vi "4Pi 4Pi Modes Control.vi"(7 "Calling VI Ref":refnum<vi>) -> ()   [LabVIEW 2016]
uses:
  <vilib>/Analysis/NI_AALBase.lvlib
  <vilib>/Utility/file.llb/Read Delimited Spreadsheet (DBL).vi
  <vilib>/Utility/miscctls.llb/LVPointTypeDef.ctl
  <vilib>/Analysis/baseanly.llb/Mean (DBL).vi
  4Pi 4Pi Modes - Controls/4Pi 4Pi Modes - Standard Action.ctl
  <vilib>/Utility/file.llb/Write Delimited Spreadsheet (DBL).vi
  4Pi 4Pi Modes - Controls/4Pi 4Pi Modes - Mirror Modes.ctl
panel:
  out "Pixel Map (-1 to 1) 2":dbl[][](graph)
  in  "Scan Modes":bool
  in  "Astig On/Off":bool
  in  "Load Astig":bool
  in  "Active Mirror":enum32{"Mirror 1", "Mirror 2"}(radio)
  in  "Clear Modes":bool
  in  "Mirror Modes":T1
  in  "Load Modes":bool
  in  "Save Modes":bool
  in  "Load Flat":bool
  in  "Apply Zero":bool
  in  "Load V Map":bool
  in  "Save V Map":bool
  in  "Apply Flat":bool
  in  "Center Bias":bool
  in  "Quit":bool
  out "Pixel Map (-1 to 1)":dbl[][](graph)
  # "Mode"
  # "Amount (nm)"
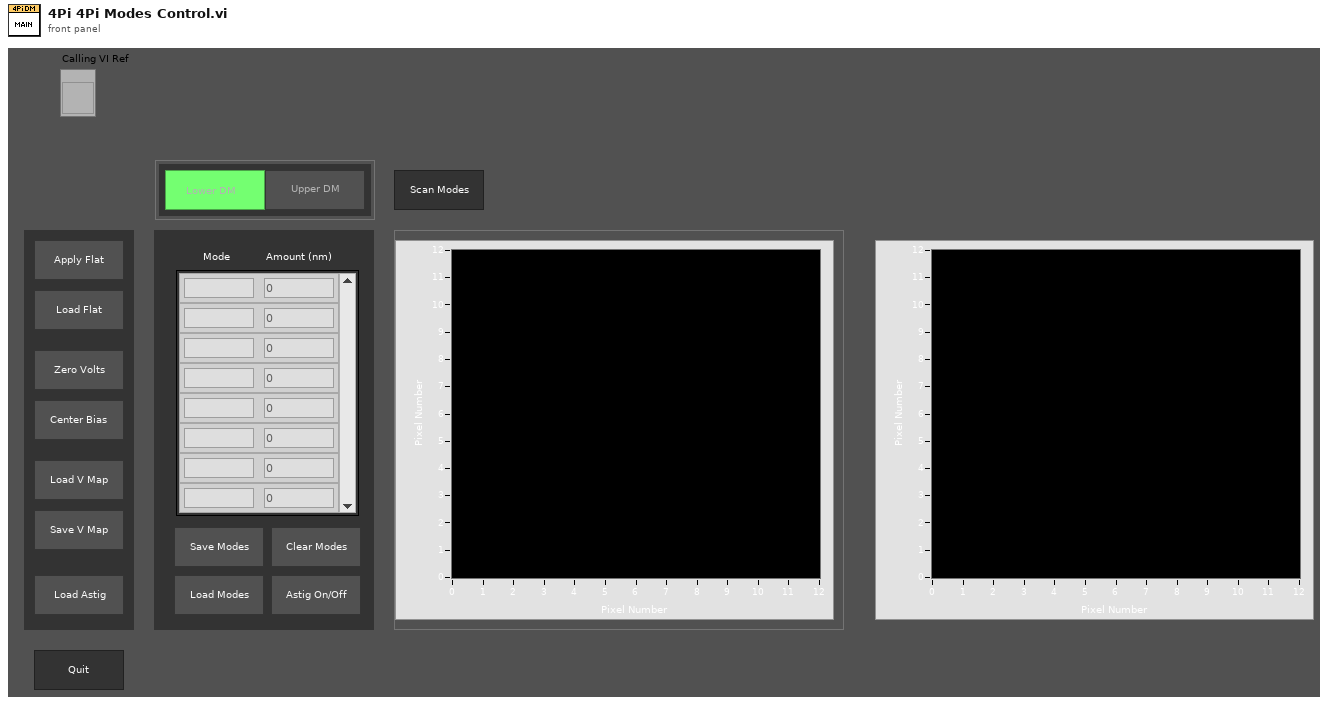
[diagram p1: front panel]
types:
  T1 = typedef "4Pi 4Pi Modes - Mirror Modes.ctl" = cluster{"Mode":string, "Amplitude":dbl}[]
  T2 = enum16{"Always On", "Always Off", "Off While Running"}
  T3 = typedef "LVPointTypeDef.ctl" = cluster{"Horizontal":i16, "Vertical":i16}
  T4 = typedef "4Pi 4Pi Modes - Standard Action.ctl" = enum16{"Read", "Write"}
  T5 = typedef "4Pi 4Pi Modes - Mirror Modes DUAL.ctl" = cluster{"Mode":string, "Amplitude":dbl}[][]
  T6 = typedef "LVRectTypeDef.ctl" = cluster{"Left":i16, "Top":i16, "Right":i16, "Bottom":i16}
  T7 = typedef "LVBoundsTypeDef.ctl" = cluster{"Width":u32, "Height":u32}
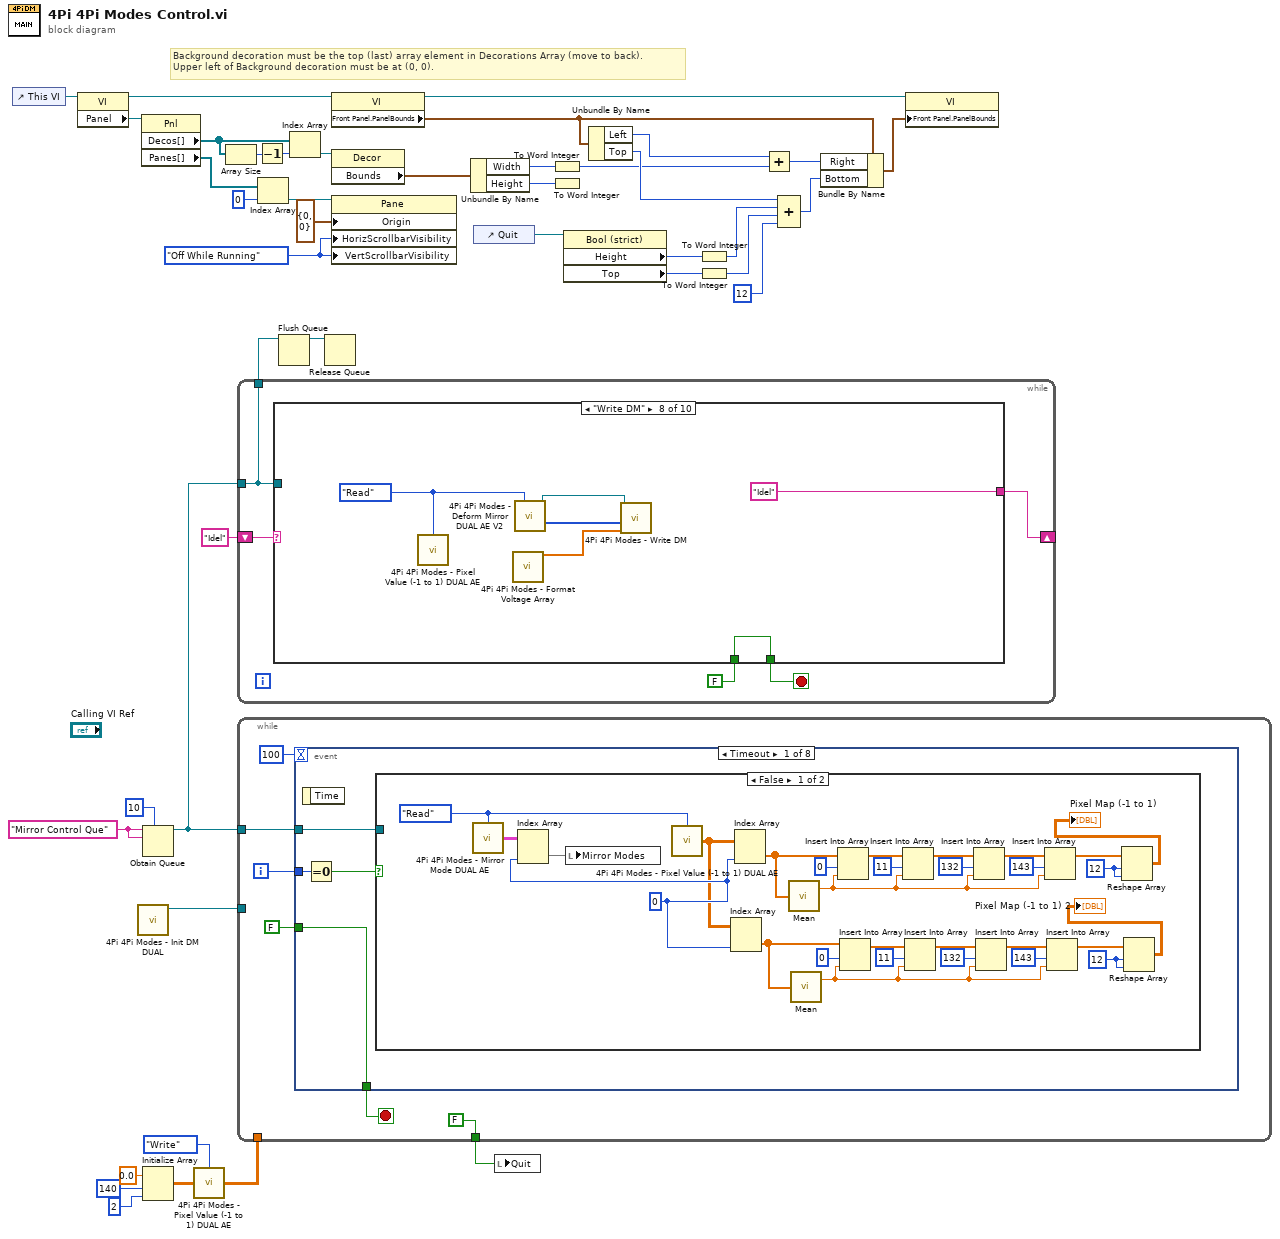
[diagram p0: block diagram]
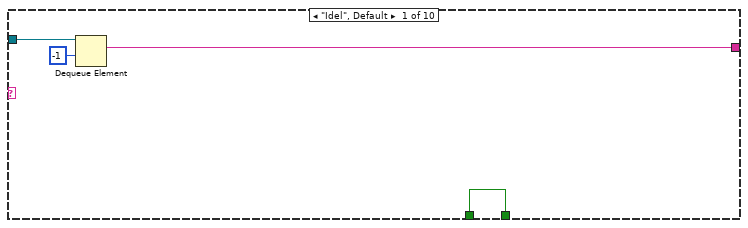
[diagram p2: hidden frame]
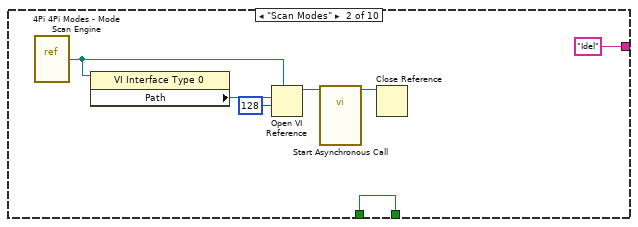
[diagram p3: hidden frame]
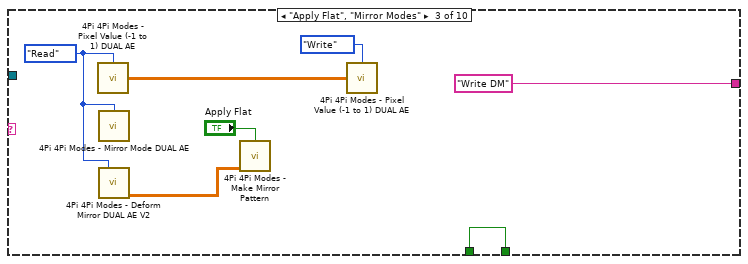
[diagram p4: hidden frame]
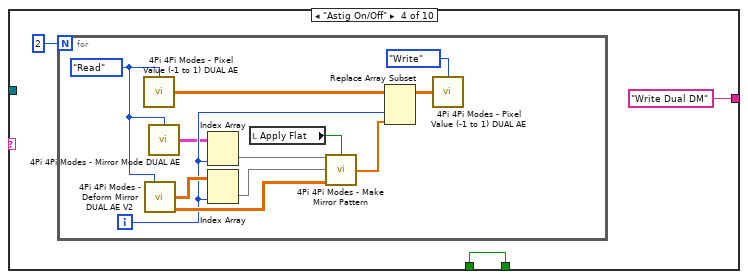
[diagram p5: hidden frame]
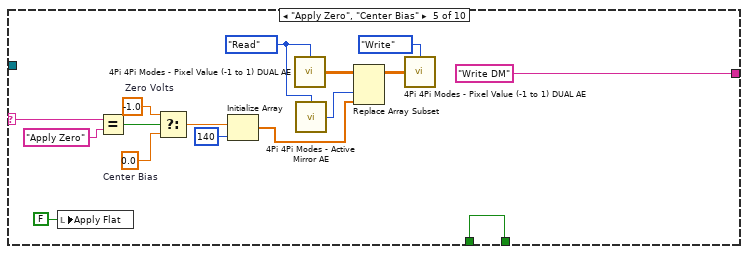
[diagram p6: hidden frame]
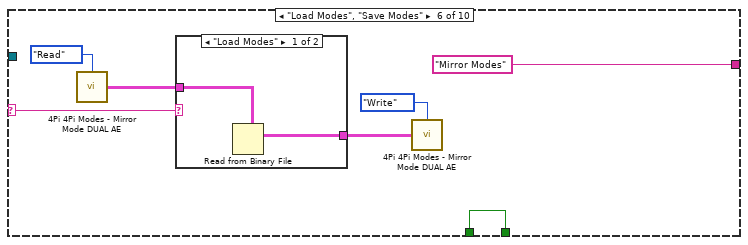
[diagram p7: hidden frame]
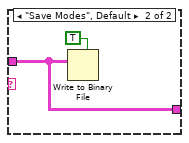
[diagram p8: hidden frame]
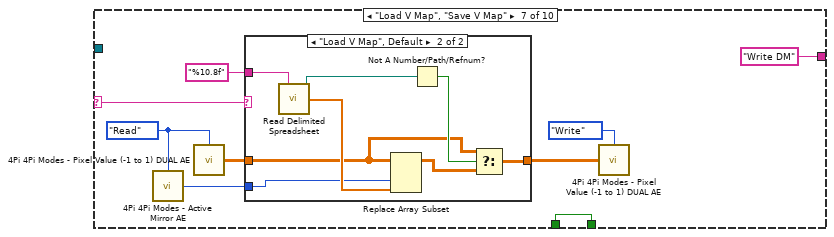
[diagram p9: hidden frame]
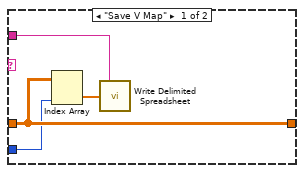
[diagram p10: hidden frame]
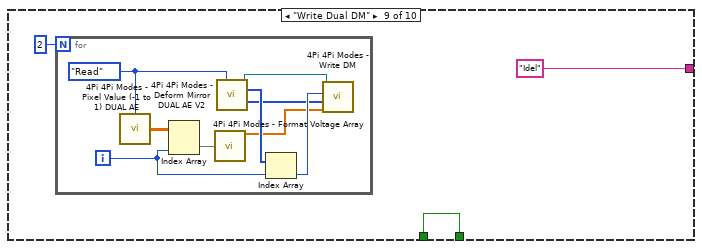
[diagram p11: hidden frame]
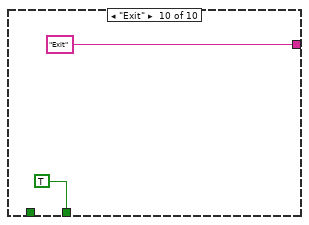
[diagram p12: hidden frame]
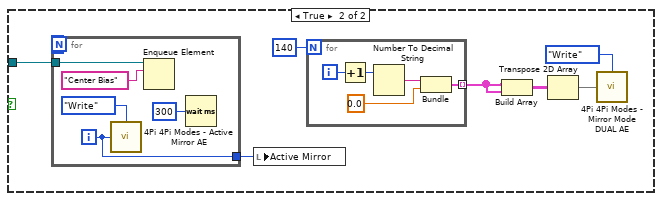
[diagram p13: hidden frame]
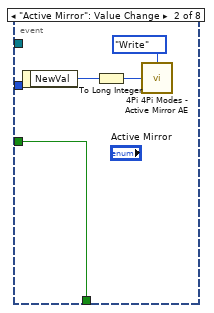
[diagram p14: hidden frame]
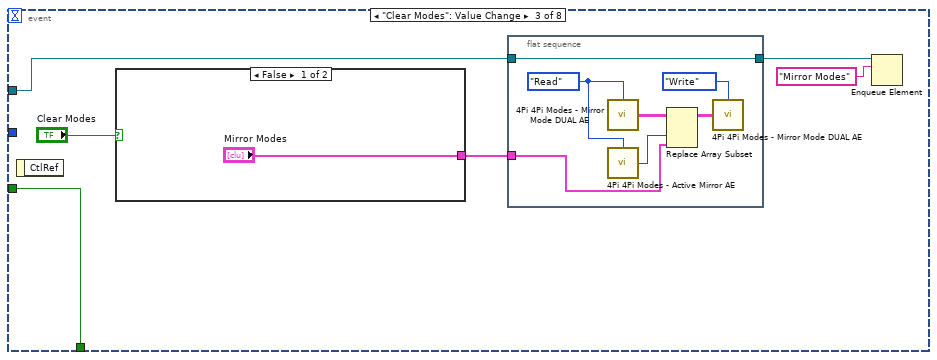
[diagram p15: hidden frame]
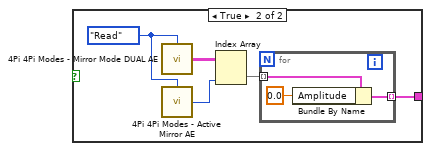
[diagram p16: hidden frame]
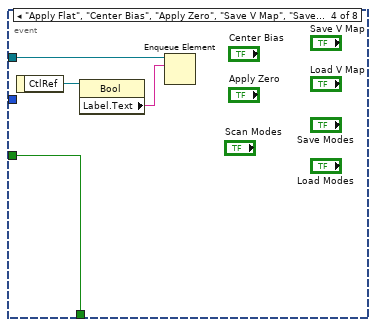
[diagram p17: hidden frame]
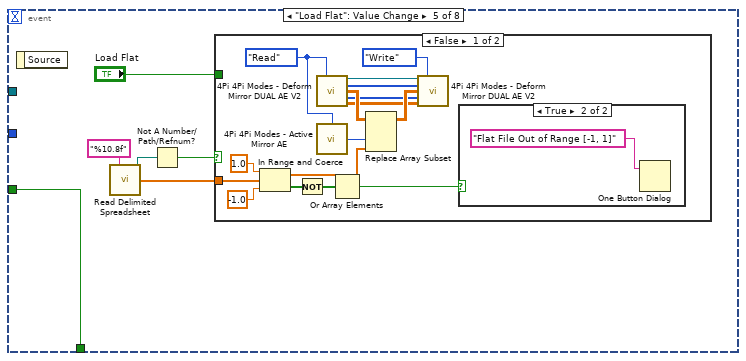
[diagram p18: hidden frame]
diagram:
  w13 = T2."Off While Running" ("Vertical Scrollbar Visibility")
  w43 = "Mirror Control Que" ("name (unnamed)")
  # "Background decoration must be the top (last) array element in Decorations Array (move to back).\nUpper left of Background decoration must be at (0, 0)."
  n1 = control-ref of="This VI"() -> (w5:refnum<vi>)
  n2 = property class="VI"(reference=w5) -> (reference out=w14:refnum<vi>, "Panel"=w6:refnum<vi>)  [unwired: 1 in, 1 out]
  n3 = call "4Pi 4Pi Modes - Init DM DUAL.vi"() -> ("reference out"=w41:refnum<k7>)  [unwired: 11 in]
  n4 = property class="Pnl"(reference=w6) -> ("Decos[]"=w4:refnum<vi>[], "Panes[]"=w10:refnum<vi>[])  [unwired: 1 in, 2 out]
  n5 = Obtain Queue(max queue size (-1, unlimited)=10, name (unnamed)=w43, element data type=w43) -> (queue out=w37:refnum<queue>)  [unwired: 2 in, 2 out]
  n6 = Initialize Array(0.0 ("element"), 140 ("dimension size"), 2 ("dimension size")) -> (w33:dbl[][])
  n7 = call "4Pi 4Pi Modes - Pixel Value (-1 to 1) DUAL AE.vi"("Action"=4Pi_4Pi_Modes_-_Standard_Action."Write", "Pixel Value (-1 to 1)"=w33) -> ("Pixel Value (-1 to 1) Out"=w31:dbl[][])  [unwired: 13 in]
  n8 = Array Size(array=w4) -> (size(s)=w2:i32)
  n9 = while {
    tunnel: w37 -> [w44]
    shift-right: [w48] -> _
    shift-left: "Idel" ("name (unnamed)") -> [w47]
    tunnel: [w44] -> w40
    stop <- w46 stop-if-true
    n10 = case shown="\"Write DM\"" w47 {
      selector: w47 -> [_ _ _ _ w93 w100 w116 _ _ _]
      tunnel: w44 -> [w52 _ _ _ _ _ _ _ _ _]
      tunnel: [w50 "Idel" ("name (unnamed)") "Write DM" ("name (unnamed)") "Write Dual DM" ("name (unnamed)") "Write DM" ("name (unnamed)") "Mirror Modes" ("name (unnamed)") "Write DM" ("name (unnamed)") "Idel" ("name (unnamed)") "Idel" ("name (unnamed)") "Exit" ("name (unnamed)")] -> w48
      tunnel: [w49 w59 w65 w68 w97 w104 w117 w135 w138 TRUE] -> w46
      tunnel: FALSE -> [w49 w59 w65 w68 w97 w104 w117 w135 w138 _]
      frame "Idel", Default {
        n11 = Dequeue Element(queue=w52, timeout in ms (-1)=-1) -> (element=w50:string)  [unwired: 1 in, 3 out]
      }
      frame "Scan Modes" {
        n12 = vi-ref "4Pi 4Pi Modes - Mode Scan Engine.vi"() -> (w53:refnum<vi>)
        n13 = property class="VI Interface Type 0"(reference=w53) -> ("Path"=w54:path)  [unwired: 1 in, 2 out]
        n14 = Open VI Reference(type specifier VI Refnum (for type only)=w53, vi path=w54, options=128) -> (vi reference=w56:refnum<vi>)  [unwired: 3 in, 1 out]
        n15 = call-by-ref "Start Asynchronous Call"(reference=w56) -> (reference out=w57:refnum<vi>)  [unwired: 17 in, 1 out]
        n16 = Close Reference(reference=w57) -> ()  [unwired: 1 in, 1 out]
      }
      frame "Apply Flat", "Mirror Modes" {
        w64 = 4Pi_4Pi_Modes_-_Standard_Action."Read" ("Action")
        n17 = call "4Pi 4Pi Modes - Pixel Value (-1 to 1) DUAL AE.vi"("Action"=w64) -> ("Pixel Value (-1 to 1) Out"=w60:dbl[][])  [unwired: 14 in]
        n18 = call "4Pi 4Pi Modes - Mirror Mode DUAL AE.vi"("Action"=w64) -> ()  [unwired: 14 in, 1 out]
        n19 = call "4Pi 4Pi Modes - Deform Mirror DUAL AE V2.vi"("Action"=w64) -> ("Mode Matrix Out"=w62:dbl[][])  [unwired: 10 in, 4 out]
        n20 = call "4Pi 4Pi Modes - Make Mirror Pattern.vi"("Flat On?"="Apply Flat", "Mirror Modes Array"=w62) -> ()  [unwired: 13 in, 1 out]
        n21 = call "4Pi 4Pi Modes - Pixel Value (-1 to 1) DUAL AE.vi"("Action"=4Pi_4Pi_Modes_-_Standard_Action."Write", "Pixel Value (-1 to 1)"=w60) -> ()  [unwired: 13 in, 1 out]
      }
      frame "Astig On/Off" {
        n22 = for {
          N: 2 -> [_]
          i -> [w72]
          w70 = 4Pi_4Pi_Modes_-_Standard_Action."Read" ("Action")
          n23 = call "4Pi 4Pi Modes - Pixel Value (-1 to 1) DUAL AE.vi"("Action"=w70) -> ("Pixel Value (-1 to 1) Out"=w76:dbl[][])  [unwired: 14 in]
          n24 = call "4Pi 4Pi Modes - Deform Mirror DUAL AE V2.vi"("Action"=w70) -> ("Flat Files Out"=w80:dbl[][], "Mode Matrix Out"=w81:dbl[][])  [unwired: 10 in, 3 out]
          n25 = call "4Pi 4Pi Modes - Mirror Mode DUAL AE.vi"("Action"=w70) -> ("Mirror Modes Out"=w71:T5)  [unwired: 14 in]
          n26 = Index Array(array=w71, index (col)=w72) -> (element=w78:cluster{"Mode":string, "Amplitude":dbl}[])  [unwired: 1 in]
          n27 = Index Array(array=w80, index (col)=w72) -> (element=w79:dbl[])  [unwired: 1 in]
          n28 = local read "Apply Flat"() -> (w73:bool)
          n29 = call "4Pi 4Pi Modes - Make Mirror Pattern.vi"("Mirror Modes In"=w78, "Flat On?"=w73, "Flat File In"=w79, "Mirror Modes Array"=w81) -> ("Pixel Value U (-1 to 1)"=w75:dbl[])  [unwired: 11 in]
          n30 = Replace Array Subset(array=w76, new element=w75, index (col)=w72) -> (w74:dbl[][])  [unwired: 1 in]
          n31 = call "4Pi 4Pi Modes - Pixel Value (-1 to 1) DUAL AE.vi"("Action"=4Pi_4Pi_Modes_-_Standard_Action."Write", "Pixel Value (-1 to 1)"=w74) -> ()  [unwired: 13 in, 1 out]
        }
      }
      frame "Apply Zero", "Center Bias" {
        w85 = 4Pi_4Pi_Modes_-_Standard_Action."Read" ("Action")
        w89 = -1.0  # Zero Volts
        w91 = 0.0  # Center Bias
        n32 = local write "Apply Flat"(FALSE ("Apply Flat")) -> ()
        n33 = Equal?(x=w93, y="Apply Zero") -> (x = y?=w92:bool)
        n34 = Select(t=w89, s=w92, f=w91) -> (s? t:f=w90:dbl)
        n35 = Initialize Array(w90, 140 ("dimension size")) -> (w82:dbl[])
        n36 = call "4Pi 4Pi Modes - Pixel Value (-1 to 1) DUAL AE.vi"("Action"=w85) -> ("Pixel Value (-1 to 1) Out"=w83:dbl[][])  [unwired: 14 in]
        n37 = call "4Pi 4Pi Modes - Active Mirror AE.vi"("Action"=w85) -> ("Active Mirror"=w84:i32)  [unwired: 14 in]
        n38 = Replace Array Subset(array=w83, new element=w82, index (col)=w84) -> (w87:dbl[][])  [unwired: 1 in]
        n39 = call "4Pi 4Pi Modes - Pixel Value (-1 to 1) DUAL AE.vi"("Action"=4Pi_4Pi_Modes_-_Standard_Action."Write", "Pixel Value (-1 to 1)"=w87) -> ()  [unwired: 13 in, 1 out]
      }
      frame "Load Modes", "Save Modes" {
        n40 = call "4Pi 4Pi Modes - Mirror Mode DUAL AE.vi"("Action"=4Pi_4Pi_Modes_-_Standard_Action."Read") -> ("Mirror Modes Out"=w99:T5)  [unwired: 14 in]
        n41 = case shown="\"Load Modes\"" w100 {
          tunnel: w99 -> [w106 w107]
          tunnel: [w105 w107] -> w98
          frame "Load Modes" {
            n42 = Read from Binary File(5:w106) -> (2:w105:T5)  [unwired: 5 in, 3 out]
          }
          frame "Save Modes", Default {
            n43 = Write to Binary File(data=w107, 5:TRUE ("prepend array or string size? (T)")) -> ()  [unwired: 4 in, 3 out]
          }
        }
        n44 = call "4Pi 4Pi Modes - Mirror Mode DUAL AE.vi"("Action"=4Pi_4Pi_Modes_-_Standard_Action."Write", "Mirror Modes In"=w98) -> ()  [unwired: 13 in, 1 out]
      }
      frame "Load V Map", "Save V Map" {
        w110 = 4Pi_4Pi_Modes_-_Standard_Action."Read" ("Action")
        n45 = call "4Pi 4Pi Modes - Active Mirror AE.vi"("Action"=w110) -> ("Active Mirror"=w109:i32)  [unwired: 14 in]
        n46 = call "4Pi 4Pi Modes - Pixel Value (-1 to 1) DUAL AE.vi"("Action"=w110) -> ("Pixel Value (-1 to 1) Out"=w114:dbl[][])  [unwired: 14 in]
        n47 = case shown="\"Load V Map\", Default" w116 {
          tunnel: w114 -> [w120 w122]
          tunnel: "%10.8f" -> [w121 w129]
          tunnel: [w120 w126] -> w111
          tunnel: w109 -> [w118 w123]
          frame "Save V Map" {
            n48 = Index Array(array=w120, index (col)=w118) -> (element=w119:dbl[])  [unwired: 1 in]
            n49 = call-poly <vilib>:"Write Delimited Spreadsheet.vi"("format (%.3f)"=w121, "1D data"=w119) -> ()  [unwired: 12 in, 2 out]
          }
          frame "Load V Map", Default {
            n50 = call-poly <vilib>:"Read Delimited Spreadsheet.vi"("format (%.3f)"=w129) -> ("new file path (Not A Path if cancelled)"=w128:path, "first row"=w124:dbl[])  [unwired: 9 in, 4 out]
            n51 = Replace Array Subset(array=w122, new element=w124, index (col)=w123) -> (w125:dbl[][])  [unwired: 1 in]
            n52 = Not A Number/Path/Refnum?(number/path/refnum=w128) -> (NaN/Path/Refnum?=w127:bool)
            n53 = Select(t=w122, s=w127, f=w125) -> (s? t:f=w126:dbl[][])
          }
        }
        n54 = call "4Pi 4Pi Modes - Pixel Value (-1 to 1) DUAL AE.vi"("Action"=4Pi_4Pi_Modes_-_Standard_Action."Write", "Pixel Value (-1 to 1)"=w111) -> ()  [unwired: 13 in, 1 out]
      }
      frame "Write DM" {
        w130 = 4Pi_4Pi_Modes_-_Standard_Action."Read" ("Action")
        n55 = call "4Pi 4Pi Modes - Pixel Value (-1 to 1) DUAL AE.vi"("Action"=w130) -> ()  [unwired: 14 in, 1 out]
        n56 = call "4Pi 4Pi Modes - Format Voltage Array.vi"() -> ("Voltage Array (Volts)"=w131:dbl[])  [unwired: 14 in, 1 out]
        n57 = call "4Pi 4Pi Modes - Deform Mirror DUAL AE V2.vi"("Action"=w130) -> ("Refnum Out"=w133:refnum<k7>, "Multi Map Data Out"=w132:i32[])  [unwired: 10 in, 3 out]
        n58 = call "4Pi 4Pi Modes - Write DM.vi"("error in (no error)"=w133, 2:w132, 3:w131) -> ()  [unwired: 4 in, 1 out]
      }
      frame "Write Dual DM" {
        n59 = for {
          N: 2 -> [_]
          i -> [w139]
          w145 = 4Pi_4Pi_Modes_-_Standard_Action."Read" ("Action")
          n60 = call "4Pi 4Pi Modes - Pixel Value (-1 to 1) DUAL AE.vi"("Action"=w145) -> ("Pixel Value (-1 to 1) Out"=w143:dbl[][])  [unwired: 14 in]
          n61 = Index Array(array=w143, index (col)=w139) -> (element=w144:dbl[])  [unwired: 1 in]
          n62 = call "4Pi 4Pi Modes - Format Voltage Array.vi"("Pixel Level (-1 to 1)"=w144) -> ("Voltage Array (Volts)"=w142:dbl[])  [unwired: 13 in, 1 out]
          n63 = call "4Pi 4Pi Modes - Deform Mirror DUAL AE V2.vi"("Action"=w145) -> ("Refnum Out"=w140:refnum<k7>, "IDs Out"=w146:i32[], "Multi Map Data Out"=w141:i32[])  [unwired: 10 in, 2 out]
          n64 = Index Array(array=w146, index=w139) -> (element=w147:i32)
          n65 = call "4Pi 4Pi Modes - Write DM.vi"("error in (no error)"=w140, 1:w147, 2:w141, 3:w142) -> ()  [unwired: 3 in, 1 out]
        }
      }
      frame "Exit" {
      }
    }
  }
  n66 = while {
    tunnel: w37 -> [w151]
    tunnel: w41 -> [_]
    tunnel: w31 -> [_]
    tunnel: [FALSE] -> w1
    i -> [w152]
    stop <- w155 stop-if-true
    n67 = event shown="[0] Timeout" {
      selector: _ -> [_ _ _ _ _ _ _ _]
      dyn-events: _ -> [_ _ _ _ _ _ _ _]
      timeout: 100 -> [_ _ _ _ _ _ _ _]
      tunnel: [w159 w210 w216 w236 w242 w264 w268 w297] -> w155
      tunnel: FALSE -> [w159 w210 w216 w236 w242 w264 w268 _]
      tunnel: w152 -> [w158 _ _ _ _ _ _ _]
      tunnel: w151 -> [w156 _ w215 w235 _ _ w265 w295]
      event Timeout {
        n68 = event-data() -> ()  [unwired: 1 in, 1 out]
        n69 = Equal To 0?(x=w158) -> (x = 0?=w157:bool)
        n70 = case shown="False" w157 {
          tunnel: w156 -> [_ w196]
          frame False {
            w162 = 0 ("index (col)")
            w173 = 12 ("dimension size")
            w186 = 12 ("dimension size")
            w187 = 4Pi_4Pi_Modes_-_Standard_Action."Read" ("Action")
            n71 = call "4Pi 4Pi Modes - Mirror Mode DUAL AE.vi"("Action"=w187) -> ("Mirror Modes Out"=w174:T5)  [unwired: 14 in]
            n72 = Index Array(array=w174, index (col)=w162) -> (element=w175:cluster{"Mode":string, "Amplitude":dbl}[])  [unwired: 1 in]
            n73 = local write "Mirror Modes"(w175) -> ()
            n74 = call "4Pi 4Pi Modes - Pixel Value (-1 to 1) DUAL AE.vi"("Action"=w187) -> ("Pixel Value (-1 to 1) Out"=w161:dbl[][])  [unwired: 14 in]
            n75 = Index Array(array=w161, index (col)=w162) -> (element=w160:dbl[])  [unwired: 1 in]
            n76 = Index Array(array=w161, index (col)=w162) -> (element=w188:dbl[])  [unwired: 1 in]
            n77 = call-poly <vilib>:"Mean.vi"("X"=w188) -> ("mean"=w184:dbl)  [unwired: 1 out]
            n78 = call-poly <vilib>:"Mean.vi"("X"=w160) -> ("mean"=w172:dbl)  [unwired: 1 out]
            n79 = Insert Into Array(array=w188, index=0, new element=w184) -> (w179:dbl[])
            n80 = Insert Into Array(array=w160, index=0, new element=w172) -> (w167:dbl[])
            n81 = Insert Into Array(array=w179, index=11, new element=w184) -> (w181:dbl[])
            n82 = Insert Into Array(array=w167, index=11, new element=w172) -> (w169:dbl[])
            n83 = Insert Into Array(array=w181, index=132, new element=w184) -> (w183:dbl[])
            n84 = Insert Into Array(array=w169, index=132, new element=w172) -> (w171:dbl[])
            n85 = Insert Into Array(array=w183, index=143, new element=w184) -> (w176:dbl[])
            n86 = Insert Into Array(array=w171, index=143, new element=w172) -> (w164:dbl[])
            n87 = Reshape Array(w176, w186, w186) -> (→"Pixel Map (-1 to 1)":dbl[][])
            n88 = Reshape Array(w164, w173, w173) -> (→"Pixel Map (-1 to 1) 2":dbl[][])
          }
          frame True {
            n89 = for {
              N: 2 -> [_]
              tunnel: w196 -> [w201]
              tunnel: [w197] -> w189
              i -> [w197]
              n90 = call "4Pi 4Pi Modes - Active Mirror AE.vi"("Action"=4Pi_4Pi_Modes_-_Standard_Action."Write", "Active Mirror In"=w197) -> ()  [unwired: 13 in, 1 out]
              n91 = Enqueue Element(queue=w201, element="Center Bias") -> ()  [unwired: 2 in, 3 out]
              n92 = Wait (ms)(milliseconds to wait=u32 300) -> ()  [unwired: 1 out]
            }
            n93 = local write "Active Mirror"(w189) -> ()
            n94 = for {
              N: 140 -> [_]
              tunnel: [w202] -> w193 mode=indexing
              i -> [w206]
              n95 = Increment(x=w206) -> (x+1=w205:i32)
              n96 = Number To Decimal String(number=w205) -> (decimal integer string=w204:string)  [unwired: 1 in]
              n97 = Bundle(w204, 0.0) -> (w202:cluster{string, dbl})  [unwired: 1 in]
            }
            n98 = Build Array(w193, w193) -> (w191:cluster{string, dbl}[][])
            n99 = Transpose 2D Array(2D array=w191) -> (transposed array=w190:cluster{string, dbl}[][])
            n100 = call "4Pi 4Pi Modes - Mirror Mode DUAL AE.vi"("Action"=4Pi_4Pi_Modes_-_Standard_Action."Write", "Mirror Modes In"=w190) -> ()  [unwired: 13 in, 1 out]
          }
        }
      }
      event "Active Mirror": Value Change {
        n101 = event-data() -> ("NewVal"=w209:enum32{"Mirror 1", "Mirror 2"})  [unwired: 1 in]
        n102 = To Long Integer(number=w209) -> (32bit integer=w208:i32)
        n103 = call "4Pi 4Pi Modes - Active Mirror AE.vi"("Action"=4Pi_4Pi_Modes_-_Standard_Action."Write", "Active Mirror In"=w208) -> ()  [unwired: 13 in, 1 out]
      }
      event "Clear Modes": Value Change {
        n104 = event-data() -> ()  [unwired: 1 in, 1 out]
        n105 = case shown="False" "Clear Modes" {
          tunnel: ["Mirror Modes" w218] -> w211
          frame False {
          }
          frame True {
            w221 = 4Pi_4Pi_Modes_-_Standard_Action."Read" ("Action")
            n106 = call "4Pi 4Pi Modes - Mirror Mode DUAL AE.vi"("Action"=w221) -> ("Mirror Modes Out"=w220:T5)  [unwired: 14 in]
            n107 = call "4Pi 4Pi Modes - Active Mirror AE.vi"("Action"=w221) -> ("Active Mirror"=w222:i32)  [unwired: 14 in]
            n108 = Index Array(array=w220, index (col)=w222) -> (element=w219:cluster{"Mode":string, "Amplitude":dbl}[])  [unwired: 1 in]
            n109 = for {
              tunnel: w219 -> [w225] mode=indexing
              tunnel: [w223] -> w218 mode=indexing
              n110 = Bundle By Name(cluster=w225, "Amplitude"=0.0) -> (w223:cluster{"Mode":string, "Amplitude":dbl})
            }
          }
        }
        n111 = flat-sequence {
          tunnel: w211 -> [w226]
          tunnel: w215 -> [w232]
          tunnel: [w232] -> w213
          frame #0 {
            w229 = 4Pi_4Pi_Modes_-_Standard_Action."Read" ("Action")
            n112 = call "4Pi 4Pi Modes - Mirror Mode DUAL AE.vi"("Action"=w229) -> ("Mirror Modes Out"=w228:T5)  [unwired: 14 in]
            n113 = call "4Pi 4Pi Modes - Active Mirror AE.vi"("Action"=w229) -> ("Active Mirror"=w230:i32)  [unwired: 14 in]
            n114 = Replace Array Subset(array=w228, new element=w226, index (col)=w230) -> (w231:T5)  [unwired: 1 in]
            n115 = call "4Pi 4Pi Modes - Mirror Mode DUAL AE.vi"("Action"=4Pi_4Pi_Modes_-_Standard_Action."Write", "Mirror Modes In"=w231) -> ()  [unwired: 13 in, 1 out]
          }
        }
        n116 = Enqueue Element(queue=w213, element="Mirror Modes") -> ()  [unwired: 2 in, 3 out]
      }
      event "Apply Flat", "Center Bias", "Apply Zero", "Save V Map", "Save Modes", "Load Modes", "Load V Map", "Scan Modes": Value Change {
        n117 = event-data() -> ("CtlRef"=w234:refnum<vi>)  [unwired: 1 in]
        n118 = property class="Bool"(reference=w234) -> ("Label.Text"=w233:string)  [unwired: 1 in, 2 out]
        n119 = Enqueue Element(queue=w235, element=w233) -> ()  [unwired: 2 in, 3 out]
      }
      event "Load Flat": Value Change {
        n120 = event-data() -> ()  [unwired: 1 in, 1 out]
        n121 = call-poly <vilib>:"Read Delimited Spreadsheet.vi"("format (%.3f)"="%10.8f") -> ("new file path (Not A Path if cancelled)"=w240:path, "first row"=w238:dbl[])  [unwired: 9 in, 4 out]
        n122 = Not A Number/Path/Refnum?(number/path/refnum=w240) -> (NaN/Path/Refnum?=w239:bool)
        n123 = case shown="False" w239 {
          tunnel: w238 -> [w258 _]
          tunnel: "Load Flat" -> [_ _]
          frame False {
            w249 = 4Pi_4Pi_Modes_-_Standard_Action."Read" ("Action")
            n124 = In Range and Coerce(upper limit=1.0, x=w258, lower limit=-1.0) -> (coerced(x)=w243:dbl[], In Range?=w255:bool[])
            n125 = Not(x=w255) -> (.not. x?=w254:bool[])
            n126 = call "4Pi 4Pi Modes - Deform Mirror DUAL AE V2.vi"("Action"=w249) -> ("Refnum Out"=w244:refnum<k7>, "IDs Out"=w245:i32[], "Flat Files Out"=w250:dbl[][], "Multi Map Data Out"=w246:i32[], "Mode Matrix Out"=w247:dbl[][])  [unwired: 10 in]
            n127 = call "4Pi 4Pi Modes - Active Mirror AE.vi"("Action"=w249) -> ("Active Mirror"=w252:i32)  [unwired: 14 in]
            n128 = Or Array Elements(Boolean array=w254) -> (logical OR=w253:bool)
            n129 = Replace Array Subset(array=w250, new element=w243, index (col)=w252) -> (w251:dbl[][])  [unwired: 1 in]
            n130 = call "4Pi 4Pi Modes - Deform Mirror DUAL AE V2.vi"("Refnum In"=w244, "Action"=4Pi_4Pi_Modes_-_Standard_Action."Write", "IDs In"=w245, "Flat Files In"=w251, "Multi Map Data In"=w246, "Mode Matrix"=w247) -> ()  [unwired: 5 in, 5 out]
            n131 = case shown="True" w253 {
              frame False {
              }
              frame True {
                n132 = One Button Dialog(message="Flat File Out of Range [-1, 1]") -> ()  [unwired: 1 in, 1 out]
              }
            }
          }
          frame True {
          }
        }
      }
      event "Load Astig": Value Change {
        n133 = event-data() -> ()  [unwired: 1 in, 1 out]
        n134 = call "4Pi 4Pi Modes - Astig Modes AE.vi"("Action"=4Pi_4Pi_Modes_-_Standard_Action."Read") -> ("Mirror Modes Out"=w263:T5)  [unwired: 14 in]
        n135 = Read from Binary File(5:w263) -> (2:w260:T5)  [unwired: 5 in, 3 out]
        n136 = call "4Pi 4Pi Modes - Astig Modes AE.vi"("Action"=4Pi_4Pi_Modes_-_Standard_Action."Write", "Mirror Modes In"=w260) -> ()  [unwired: 13 in, 1 out]
      }
      event "Astig On/Off": Value Change {
        n137 = event-data() -> ()  [unwired: 1 in, 1 out]
        n138 = case shown="True" "Astig On/Off" {
          tunnel: [w273 w285] -> w266
          frame False {
            n139 = for {
              N: 2 -> [_]
              tunnel: [w276] -> w274 mode=indexing
              i -> [w277]
              n140 = call "4Pi 4Pi Modes - Mirror Mode DUAL AE.vi"("Action"=4Pi_4Pi_Modes_-_Standard_Action."Read") -> ("Mirror Modes Out"=w279:T5)  [unwired: 14 in]
              n141 = Index Array(array=w279, index (col)=w277) -> (element=w280:cluster{"Mode":string, "Amplitude":dbl}[])  [unwired: 1 in]
              n142 = for {
                tunnel: w280 -> [w283] mode=indexing
                tunnel: [w281] -> w276 mode=indexing
                n143 = Bundle By Name(cluster=w283, "Amplitude"=0.0) -> (w281:cluster{"Mode":string, "Amplitude":dbl})
              }
            }
            n144 = Transpose 2D Array(2D array=w274) -> (transposed array=w273:cluster{"Mode":string, "Amplitude":dbl}[][])
          }
          frame True {
            n145 = call "4Pi 4Pi Modes - Astig Modes AE.vi"("Action"=4Pi_4Pi_Modes_-_Standard_Action."Read") -> ("Mirror Modes Out"=w285:T5)  [unwired: 14 in]
          }
        }
        n146 = flat-sequence {
          tunnel: w266 -> [w270]
          tunnel: w265 -> [w271]
          frame #0 {
            n147 = call "4Pi 4Pi Modes - Mirror Mode DUAL AE.vi"("Action"=4Pi_4Pi_Modes_-_Standard_Action."Write", "Mirror Modes In"=w270) -> ()  [unwired: 13 in, 1 out]
          }
          frame #1 {
            n148 = Enqueue Element(queue=w271, element="Astig On/Off") -> ()  [unwired: 2 in, 3 out]
          }
        }
      }
      event "Quit": Value Change {
        n149 = event-data() -> ("NewVal"=w297:bool)  [unwired: 1 in]
        n150 = for {
          N: 2 -> [_]
          tunnel: w295 -> [w303]
          tunnel: [w298] -> w286
          i -> [w299]
          n151 = call "4Pi 4Pi Modes - Active Mirror AE.vi"("Action"=4Pi_4Pi_Modes_-_Standard_Action."Write", "Active Mirror In"=w299) -> ()  [unwired: 13 in, 1 out]
          n152 = Enqueue Element(queue=w303, element="Apply Zero") -> (queue out=w298:refnum<queue>)  [unwired: 2 in, 2 out]
          n153 = Wait (ms)(milliseconds to wait=u32 300) -> ()  [unwired: 1 out]
        }
        n154 = Enqueue Element(queue=w286, element="Exit") -> (error out=w290:errorcluster)  [unwired: 2 in, 2 out]
        n155 = call "4Pi 4Pi Modes - Deform Mirror DUAL AE V2.vi"("Action"=4Pi_4Pi_Modes_-_Standard_Action."Read") -> ("Refnum Out"=w293:refnum<k7>, "IDs Out"=w288:i32[])  [unwired: 10 in, 3 out]
        n156 = call "4Pi 4Pi Modes - Config DM.vi"("High Voltage"=FALSE, "error in (no error)"=w290, "Dev IDs"=w288, "Automation Refnum in"=w293) -> ("error out"=w289:errorcluster, "Automation Refnum out"=w292:refnum<k7>)  [unwired: 6 in]
        n157 = Close Reference(reference=w292, error in (no error)=w289) -> ()  [unwired: 1 out]
      }
    }
  }
  n158 = Decrement(x=w2) -> (x-1=w3:i32)
  n159 = Index Array(array=w10, index=0) -> (element=w9:refnum<vi>)
  n160 = Flush Queue(queue=w40) -> (queue out=w39:refnum<queue>)  [unwired: 1 in, 2 out]
  n161 = Index Array(array=w4, index=w3) -> (element=w12:refnum<vi>)
  n162 = Release Queue(queue=w39) -> ()  [unwired: 2 in, 3 out]
  n163 = property class="VI"(reference=w14) -> (reference out=w16:refnum<vi>, "Front Panel.PanelBounds"=w17:T6)  [unwired: 1 in, 1 out]
  n164 = property class="Decor"(reference=w12) -> ("Bounds"=w15:T7)  [unwired: 1 in, 2 out]
  n165 = property class="Pane"(reference=w9, "Origin"=T3 {"Horizontal"=0, "Vertical"=0}, "HorizScrollbarVisibility"=w13, "VertScrollbarVisibility"=w13) -> ()  [unwired: 1 in, 2 out]
  n166 = Unbundle By Name(w15) -> ("Width"=w20:u32, "Height"=w23:u32)
  n167 = control-ref of="Quit"() -> (w7:refnum<vi>)
  n168 = local write "Quit"(w1) -> ()
  n169 = To Word Integer(number=w20) -> (16bit integer=w22:i16)
  n170 = To Word Integer(number=w23) -> ()  [unwired: 1 out]
  n171 = property class="Bool (strict)"(reference=w7) -> ("Height"=w25:u32, "Top"=w26:i32)  [unwired: 1 in, 2 out]
  n172 = Unbundle By Name(w17) -> ("Left"=w19:i16, "Top"=w30:i16)
  n173 = To Word Integer(number=w25) -> (16bit integer=w28:i16)
  n174 = To Word Integer(number=w26) -> (16bit integer=w29:i16)
  n175 = Add(x=w19, y=w22) -> (x+y=w21:i16)
  n176 = Compound Arithmetic op=ADD(w30, w28, w29, i16 12 ("y")) -> (w24:i16)
  n177 = Bundle By Name(cluster=w17, "Right"=w21, "Bottom"=w24) -> (w18:T6)
  n178 = property class="VI"(reference=w16, "Front Panel.PanelBounds"=w18) -> ()  [unwired: 1 in, 2 out]
